vi "generate_equidistant_steps_LV16.vi"(2 "# of steps":u32, 3 "end value":dbl, 4 "start value":dbl) -> (0 "stepsize":dbl=-40.0, 1 "array out":dbl[](array[numeric]))   [LabVIEW 2016]
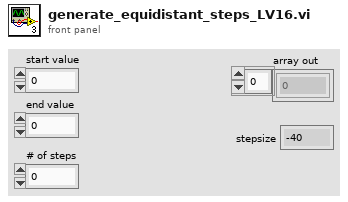
[diagram p1: front panel]
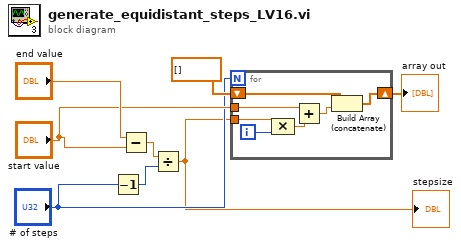
[diagram p0: block diagram]
diagram:
  n1 = Decrement(x="# of steps") -> (x-1=w3:u32)
  n2 = Subtract(x="end value", y="start value") -> (x-y=w5:dbl)
  n3 = Divide(x=w5, y=w3) -> (x/y=w2:dbl)
  "stepsize" <- w2
  n4 = for {
    N: "# of steps" -> [_]
    shift-right: [w9] -> w1
    shift-left: dbl[] [] -> [w10]
    tunnel: w2 -> [w14]
    tunnel: "start value" -> [w13]
    i -> [w15]
    n5 = Compound Arithmetic op=MULTIPLY(w14, w15) -> (w12:dbl)
    n6 = Add(x=w13, y=w12) -> (x+y=w11:dbl)
    n7 = Build Array (concatenate)(w10, w11) -> (w9:dbl[])
  }
  "array out" <- w1
